vi "configuration UI.vi"() -> ()   [LabVIEW 2013, in "Profibus Module editor node.lvclass"]
uses:
  Profibus Module editor node.lvclass
  <vilib>/NI/Configuration Framework/Node/NodeRef.ctl
  <vilib>/NI/Configuration Framework/Node/NISE_CEF_Node.lvclass
  <vilib>/NI/AMC/Message Queue.ctl
  <vilib>/NI/AMC/Message.ctl
  <vilib>/NI/Tools/Keyed Array/KeyedArray.ctl
  <vilib>/NI/Configuration Framework/Node/UserEventRef.ctl
  <vilib>/NI/Configuration Framework/Controls/EventCluster.ctl
  configuration/endianness setting.ctl
  configuration/error throw specification.ctl
  <vilib>/NI/Tag Bus Data Framework/Configuration Editor/Classes/Engine Parent/Engine Parent Editor Node.lvclass
  <vilib>/NI/Tag Bus/tag/tag descriptor.lvclass
  <vilib>/NI/Tag Bus/tag/Data Type.ctl
  <vilib>/NI/Module Execution Interface/Engine Configuration/engine configuration.lvclass
  <vilib>/NI/Tag Bus/tag/tag descriptor.lvclass/tag descriptor.ctl
  Profibus Module editor node.lvclass/Profibus Module editor node.ctl
  configuration/Profibus Module configuration.lvclass/Profibus Module configuration.ctl
  <vilib>/NI/Configuration Framework/serializable configuration/NISE_CEF_serializable configuration.lvclass/NISE_CEF_serializable configuration.ctl
  configuration/slave diagnostic configuration.ctl
  <vilib>/NI/Tag Bus Module Framework/channel/TBM channel.lvclass
  <vilib>/NI/Tag Bus/tag/write tag name.vi
  <vilib>/NI/Tag Bus/tag/write data type.vi
  configuration/Write RIO interface.vi
  <vilib>/Utility/LVClass/Get LV Class Name.vi
  <vilib>/NI/Configuration Framework/error generator/NISE_error generator.vi
  <vilib>/NI/Configuration Framework/NISE_CEF_TreeControl.lvlib
  configuration/Profibus Module configuration.lvclass
  <vilib>/NI/Tag Bus Data Framework/Configuration Editor/Classes/Module editor node/module editor node.lvclass
  channel/Profibus channel.lvclass
  <vilib>/NI/Configuration Framework/serializable configuration/NISE_CEF_serializable configuration.lvclass
  <vilib>/NI/Tools/Keyed Array/Tools_KeyedArray.lvlib
  <vilib>/NI/AMC/AMC.lvlib
panel:
  in  "Tab Control":T1(tab)
  in  "Remove Button":bool
  in  "Add Button":bool
  in  "channel":i32(listbox)
  in  "settings":bool
  in  "slave":i8
  in  "remove slave":bool
  in  "add slave":bool
  in  "byte order":T2
  out "Configured Order":T2[](array[typedef])
  in  "RIO Interface":string="RIO0"
  in  "Channel Name?":string
  in  "error specs":T3[](array[typedef])
  in  "report?":bool
  out "Selected Slave":i8
  in  "disablediag":bool
  in  "enablediag":bool
  in  "Slaves to Enable Diagnostics":i32(listbox)
  in  "Available Slaves":i32(listbox)
  in  "user event":T4
  in  "main queue":T5
  in  "node ref":T6
  # "Default configuration is little endian"
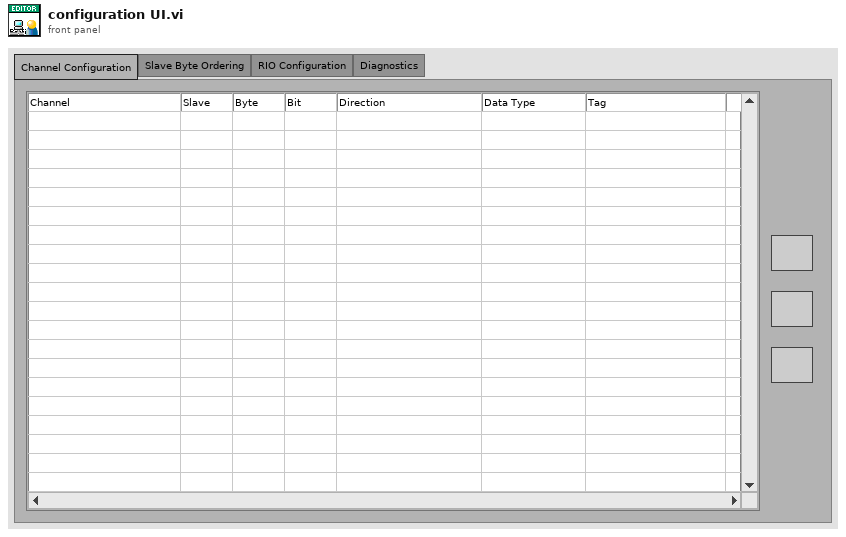
[diagram p1: front panel]
types:
  T1 = enum32{"Channel Configuration", "Slave Byte Ordering", "RIO Configuration", "Diagnostics"}
  T2 = typedef "Profibus Module configuration.lvclass/endianness setting.ctl" = cluster{"slave":i8, "big endian":bool}
  T3 = typedef "Profibus Module configuration.lvclass/error throw specification.ctl" = cluster{"byte":i32, "bit":i32, "inverted?":bool, "error":i32}
  T4 = typedef "NISE_CEF_Node.lvclass/UserEventRef.ctl" = refnum<user-event>
  T5 = typedef "AMC.lvlib/Message Queue.ctl" = refnum<queue>
  T6 = typedef "NISE_CEF_Node.lvclass/NodeRef.ctl" = refnum<data-value>
  T7 = typedef "NISE_CEF_TreeControl.lvlib/EventCluster.ctl" = cluster{"command":string, "data":string}
  T8 = typedef "tag bus.lvlib/tag descriptor.lvclass/Data Type.ctl" = enum16{"Double", "Single", "I64", "I32", "I16", "I8", "U64", "U32", "U16", "U8", "Boolean", "String", "Array of Double", "Array of Single", "Array of I64", "Array of I32", "Array of I16", "Array of I8", "Array of U64", "Array of U32", "Array of U16", "Array of U8", "Array of Boolean", "Array of String"}
  T9 = typedef "Profibus Module configuration.lvclass/slave diagnostic configuration.ctl" = cluster{"slave":i8, "report":bool, "channel":refnum<class "TBM channel.lvclass">, "error specs":T3[]}
  T10 = typedef "Profibus Module editor node.lvclass/table line.ctl" = cluster{"profchan":refnum<class "Profibus channel.lvclass">, "tag name":string}
  T11 = typedef "LVPoint32TypeDef.ctl" = cluster{"Horizontal":i32, "Vertical":i32}
  T12 = typedef "LVRowAndColumnTypeDef.ctl" = cluster{"Row":i32, "Column":i32}
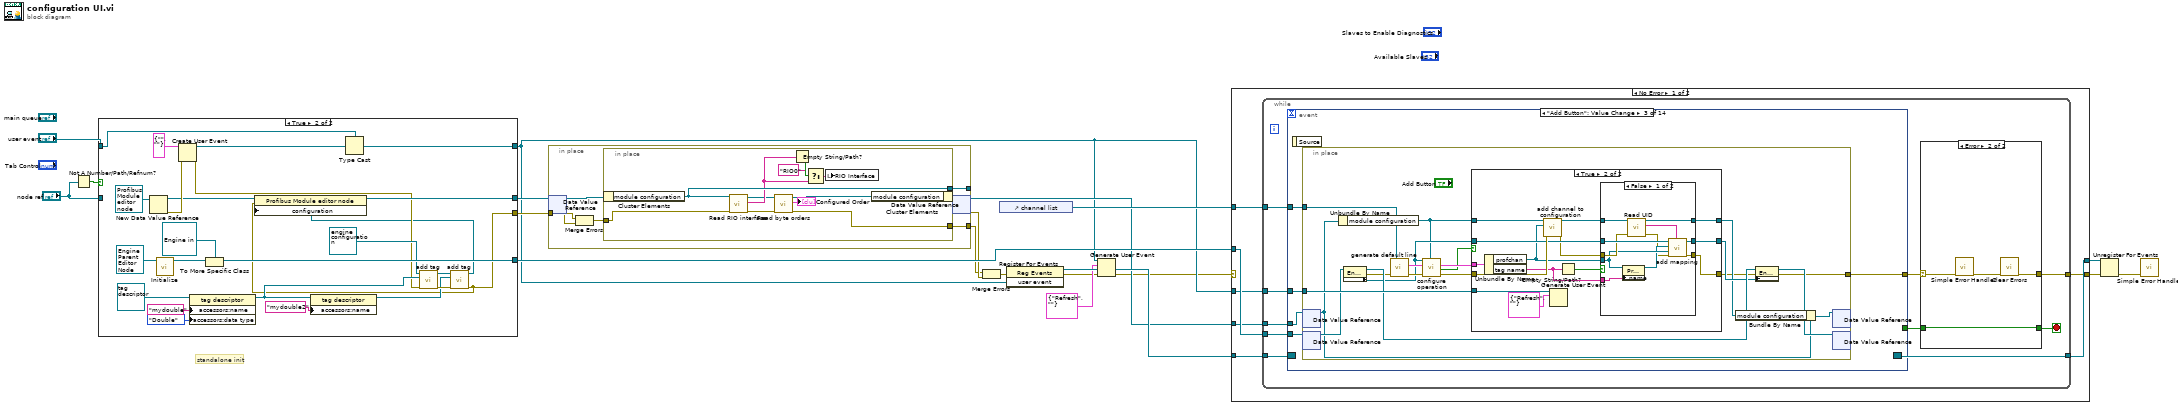
[diagram p0: block diagram]
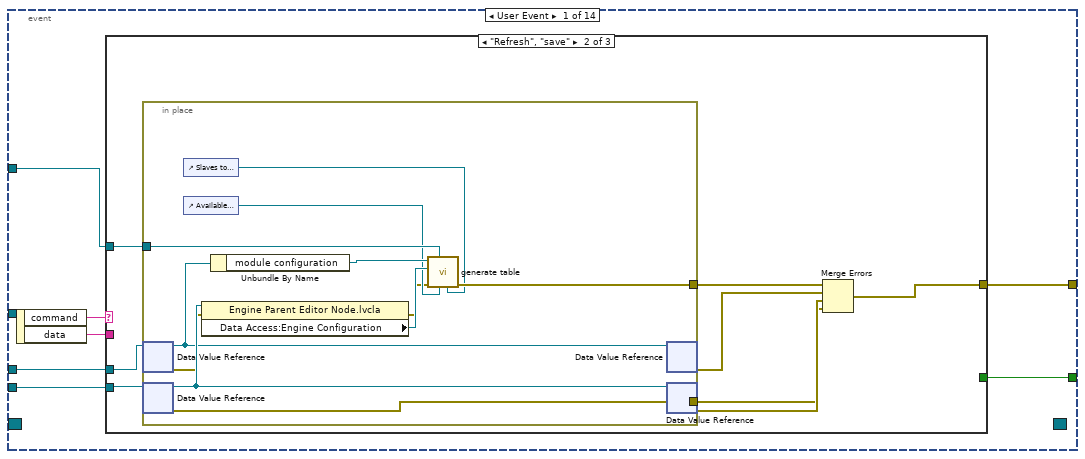
[diagram p3: hidden frame]
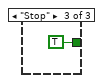
[diagram p5: hidden frame]
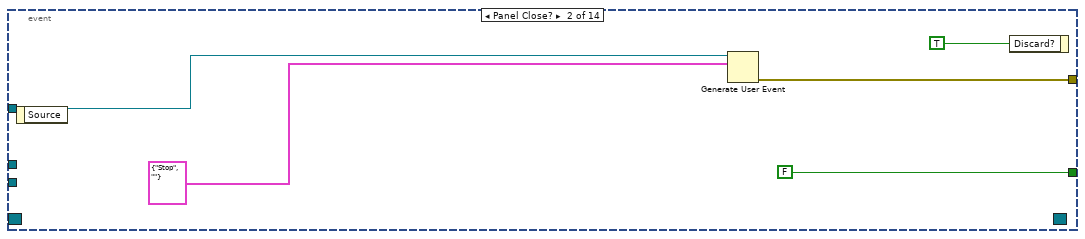
[diagram p6: hidden frame]
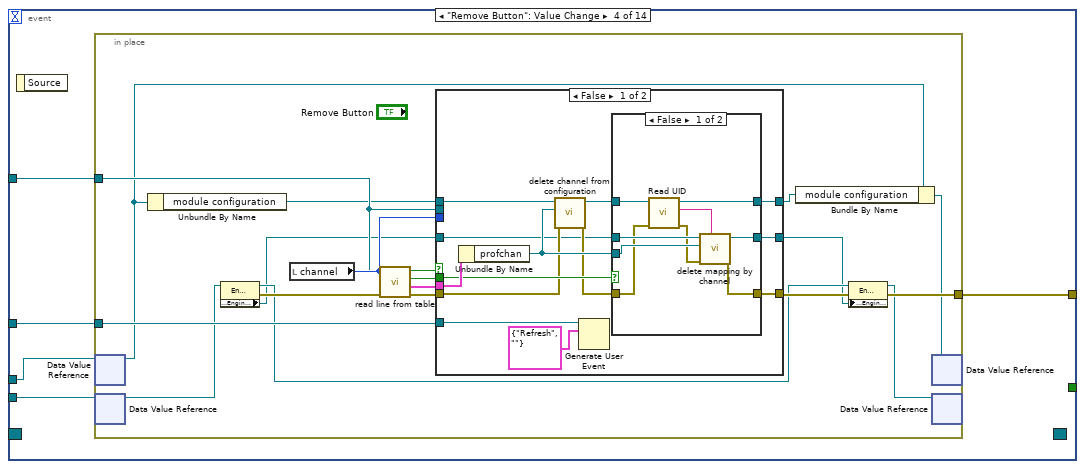
[diagram p9: hidden frame]
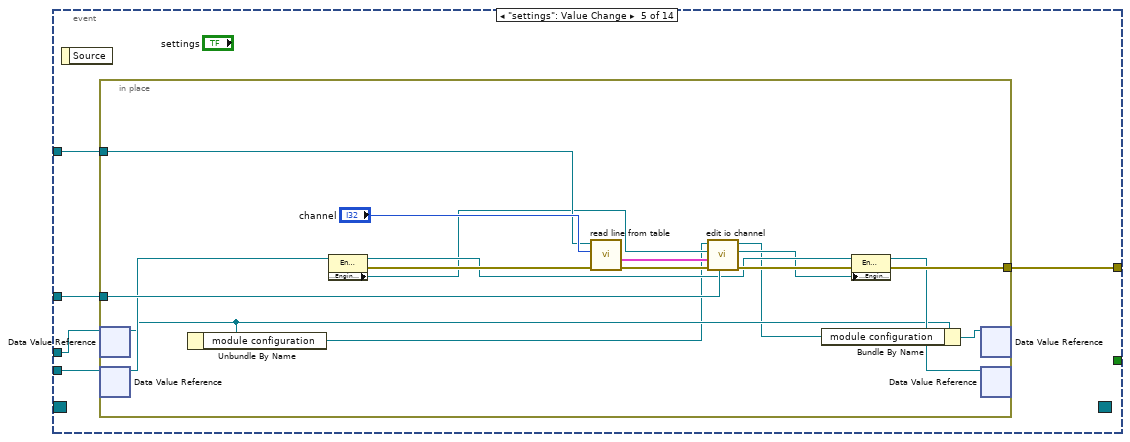
[diagram p12: hidden frame]
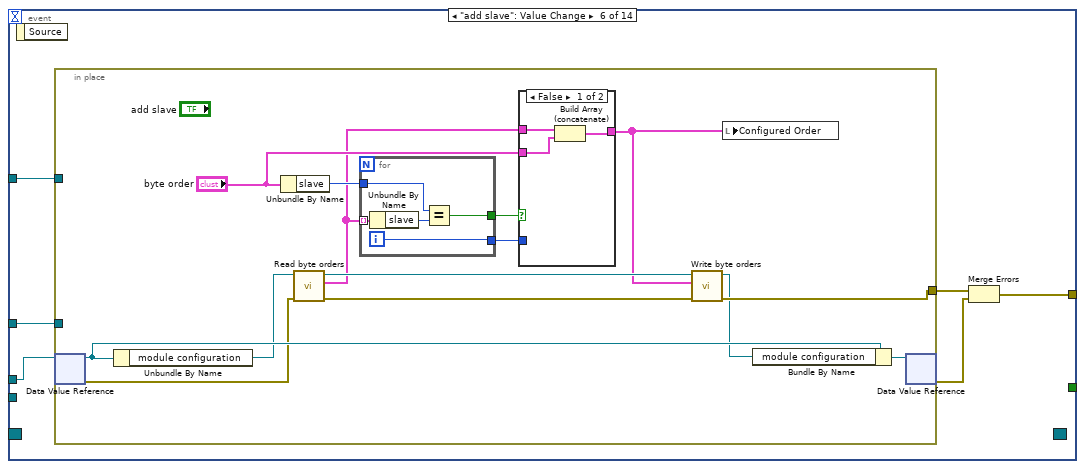
[diagram p13: hidden frame]
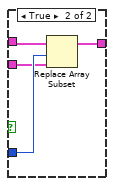
[diagram p14: hidden frame]
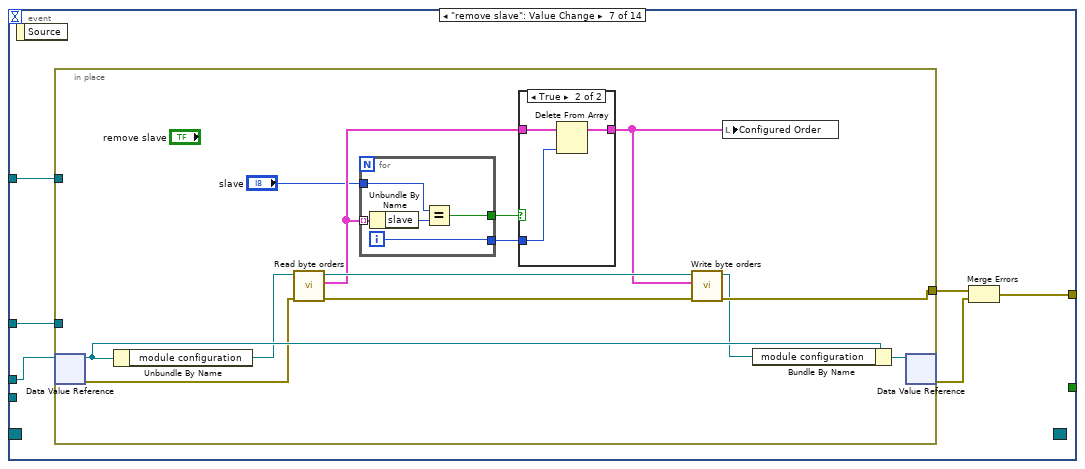
[diagram p15: hidden frame]
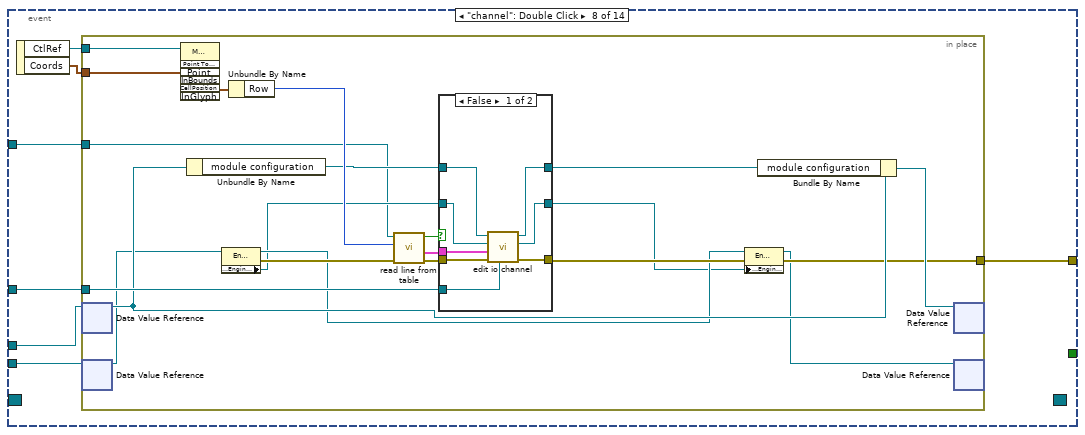
[diagram p17: hidden frame]
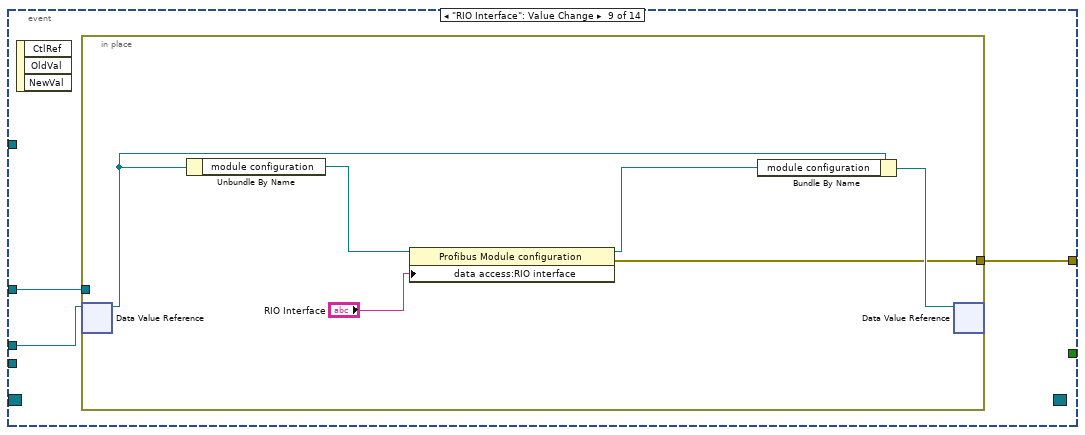
[diagram p19: hidden frame]
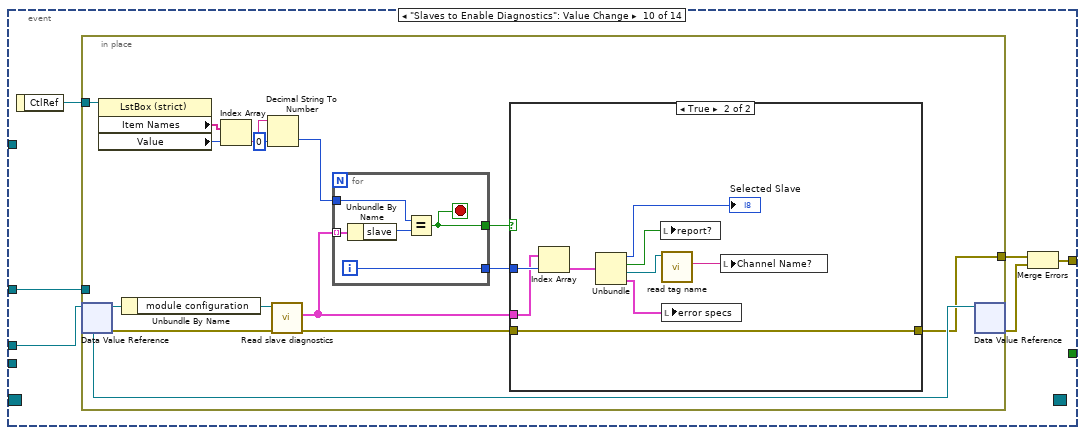
[diagram p20: hidden frame]
diagram:
  # "standalone init"
  n1 = Not A Number/Path/Refnum?(number/path/refnum="node ref") -> (NaN/Path/Refnum?=w16:bool)
  n2 = case shown="True" w16 {
    tunnel: "user event" -> [w26 w31]
    tunnel: [w26 w32] -> w3
    tunnel: "node ref" -> [w24 _]
    tunnel: [w23 w46] -> w10
    tunnel: [w22 w28] -> w9
    tunnel: [w21 w43] -> w14
    frame False {
      n3 = call <vilib>:"locate engine.vi"("component"=w24) -> ("error out"=w20:errorcluster, "engine"=w21:refnum<data-value>)  [unwired: 9 in]
      n4 = To More Specific Class(target class=refnum<data-value> refnum ("data value reference"), reference=w24, error in=w20) -> (specific class reference=w23:refnum<data-value>, error out=w22:errorcluster)
    }
    frame True {
      n5 = New Data Value Reference(data value=refnum<class "Profibus Module editor node.lvclass"> refnum ("tag bus configurable plugin editor node")) -> (data value reference=w45:refnum<data-value>, error out=w47:errorcluster)  [unwired: 1 in]
      n6 = call-dynamic "Initialize.vi"("Engine in"=refnum<class "Engine Parent Editor Node.lvclass"> refnum) -> ("data value reference"=w44:T6)  [unwired: 8 in, 2 out]
      n7 = Create User Event(user event datatype=T7 {"command"="", "data"=""} ("event data"), error in=w47) -> (user event=w49:refnum<user-event>, error out=w29:errorcluster)
      n8 = property class="tag descriptor"(reference=refnum<class "tag descriptor.lvclass"> refnum ("tag descriptor"), "accessors:name"="mydouble" ("name"), "accessors:data type"=Data_Type."Double" ("data type")) -> (reference out=w33:refnum<class "tag descriptor.lvclass">)  [unwired: 1 in, 1 out]
      n9 = To More Specific Class(target class=refnum<data-value> refnum ("data value reference"), reference=w44) -> (specific class reference=w43:refnum<data-value>)  [unwired: 1 in, 1 out]
      n10 = property class="tag descriptor"(reference=w33, "accessors:name"="mydouble2" ("name")) -> (reference out=w34:refnum<class "tag descriptor.lvclass">)  [unwired: 1 in, 1 out]
      n11 = Type Cast(type=w31, x=w49) -> (*(type *) &x=w32:T4)
      n12 = call <vilib>:"add tag.vi"("error in"=w29, "tag descriptor"=w33, "engine configuration in"=refnum<class "engine configuration.lvclass"> refnum ("Engine Configuration")) -> ("error out"=w36:errorcluster, "engine configuration out"=w35:refnum<class "engine configuration.lvclass">)  [unwired: 7 in]
      n13 = call <vilib>:"add tag.vi"("error in"=w36, "tag descriptor"=w34, "engine configuration in"=w35) -> ("error out"=w28:errorcluster, "engine configuration out"=w27:refnum<class "engine configuration.lvclass">)  [unwired: 7 in]
      n14 = property class="Profibus Module editor node"(reference=w45, error in=w28, "configuration"=w27) -> (reference out=w46:refnum<data-value>)  [unwired: 1 out]
    }
  }
  n15 = in-place {
    in-place-border: w9 -> [w57]
    in-place-border: [w52] -> w7
    in-place-border: [w51] -> _
    n16 = in-place-dvr #1(w10) -> (w55:refnum<class "Profibus Module editor node.lvclass">, w56:errorcluster)
    n17 = Merge Errors(w57, w56) -> (w53:errorcluster)
    n18 = in-place {
      in-place-border: w53 -> [w67]
      in-place-border: [w60] -> w52
      in-place-border: [w68] -> w51
      n19 = in-place-cluster #2(w55) -> ("module configuration"=w68:refnum<class "Profibus Module configuration.lvclass">)
      n20 = call "Read RIO interface.vi"("error in"=w67, "Profibus Module configuration in"=w68) -> ("error out"=w59:errorcluster, "RIO interface"=w63:string, "Profibus Module configuration out"=w62:refnum<class "Profibus Module configuration.lvclass">)  [unwired: 7 in]
      n21 = call "Read byte orders.vi"("error in"=w59, "Profibus Module configuration in"=w62) -> ("error out"=w60:errorcluster, "byte orders"=→"Configured Order":T2[], "Profibus Module configuration out"=w61:refnum<class "Profibus Module configuration.lvclass">)  [unwired: 7 in]
      n22 = Empty String/Path?(string/path=w63) -> (empty?=w66:bool)
      n23 = Select(t="RIO0", s=w66, f=w63) -> (s? t:f=w64:string)
      n24 = local write "RIO Interface"(w64) -> ()
      n25 = in-place-cluster #2("module configuration"=w61) -> (w54:refnum<class "Profibus Module editor node.lvclass">)
    }
    n26 = in-place-dvr #1(w54) -> (w6:refnum<data-value>, w8:errorcluster)
  }
  n27 = Merge Errors(w7, w8) -> (w5:errorcluster)
  n28 = control-ref of="channel list"() -> (w12:refnum<vi>)
  n29 = register-events(error in=w5, w3) -> (reference out=w19:refnum<event-registration>, error out=w2:errorcluster)  [unwired: 1 in]
  n30 = Generate User Event(user event=w3, event data cluster=T7 {"command"="Refresh", "data"=""} ("event data"), error in=w2) -> (error out=w1:errorcluster)  [unwired: 1 in, 1 out]
  n31 = case shown="No Error" w1 {
    selector: w1 -> [_ w546]
    tunnel: w19 -> [w75 w545]
    tunnel: [w74 w545] -> w18
    tunnel: [w73 w546] -> w17
    tunnel: w14 -> [w72 _]
    tunnel: w12 -> [w71 _]
    tunnel: w6 -> [w70 _]
    tunnel: w3 -> [w69 _]
    frame No Error {
      n32 = while {
        tunnel: w75 -> [w85]
        tunnel: [w84] -> w74
        tunnel: w70 -> [w81]
        tunnel: w72 -> [w80]
        tunnel: w69 -> [w79]
        tunnel: w71 -> [w77]
        tunnel: [w82] -> w73
        stop <- w83 stop-if-true
        n33 = event shown="[2] \"Add Button\": Value Change" {
          selector: w85 -> [_ _ _ _ _ _ _ _ _ _ _ _ _ _]
          dyn-events: [_ _ _ _ _ _ _ _ _ _ _ _ _ _] -> w84
          timeout: _ -> [_ _ _ _ _ _ _ _ _ _ _ _ _ _]
          tunnel: [w98 FALSE _ _ _ _ _ _ _ _ _ _ _ _] -> w76
          tunnel: [w93 w119 w128 w183 w234 w255 w287 w319 w354 w363 w405 w431 w467 w504] -> w78
          tunnel: w81 -> [w96 _ w124 w179 w231 w256 w288 w314 w352 w365 w406 w432 w470 w507]
          tunnel: w80 -> [w95 _ w125 w180 w232 _ _ w315 _ _ w402 _ _ _]
          tunnel: w79 -> [_ w121 w127 w182 w235 w258 w290 w318 w353 w366 w407 w433 w471 w508]
          tunnel: w77 -> [w92 _ w126 w181 w233 w257 w289 w313 _ _ _ _ _ _]
          event User Event {
            n34 = event-data() -> ("command"=w97:string, "data"=w94:string)  [unwired: 1 in]
            n35 = case shown="\"Refresh\", \"save\"" w97 {
              tunnel: [_ _ TRUE] -> w98
              tunnel: w96 -> [_ w103 _]
              tunnel: w95 -> [_ w104 _]
              tunnel: w94 -> [_ _ _]
              tunnel: [_ w102 _] -> w93
              tunnel: w92 -> [_ w105 _]
              frame Default {
              }
              frame "Refresh", "save" {
                n36 = in-place {
                  in-place-border: [w117] -> w106
                  in-place-border: w105 -> [w116]
                  in-place-border: [w107] -> w99
                  n37 = in-place-dvr #3(w103) -> (w112:refnum<class "Profibus Module editor node.lvclass">, w108:errorcluster)
                  n38 = in-place-dvr #4(w104) -> (w113:refnum<class "Engine Parent Editor Node.lvclass">, w107:errorcluster)
                  n39 = control-ref of="Slaves to Enable Diagnostics"() -> (w111:refnum<vi>)
                  n40 = control-ref of="Available Slaves"() -> (w110:refnum<vi>)
                  n41 = property class="Engine Parent Editor Node.lvcla"(reference=w113, error in=w108) -> (error out=w109:errorcluster, "Data Access:Engine Configuration"=w114:refnum<class "engine configuration.lvclass">)  [unwired: 1 out]
                  n42 = Unbundle By Name(w112) -> ("module configuration"=w115:refnum<class "Profibus Module configuration.lvclass">)
                  n43 = call "generate table.vi"("Slaves to Enable Diagnostics"=w111, "Available Slaves"=w110, "table"=w116, "error in"=w109, "engine configuration in"=w114, "Profibus Module configuration in"=w115) -> ("error out"=w117:errorcluster)  [unwired: 5 in]
                  n44 = in-place-dvr #3(w112) -> (w101:errorcluster)  [unwired: 1 out]
                  n45 = in-place-dvr #4(w113) -> (w100:errorcluster)  [unwired: 1 out]
                }
                n46 = Merge Errors(w106, w101, w100, w99) -> (w102:errorcluster)
              }
              frame "Stop" {
              }
            }
          }
          event Panel Close? {
            n47 = event-data() -> ()  [unwired: 1 in, 1 out]
            n48 = Generate User Event(user event=w121, event data cluster=T7 {"command"="Stop", "data"=""} ("event data")) -> (error out=w119:errorcluster)  [unwired: 2 in, 1 out]
            n49 = event-data("Discard?"=TRUE) -> ()  [unwired: 1 in, 1 out]
          }
          event "Add Button": Value Change {
            n50 = event-data() -> ()  [unwired: 1 in, 1 out]
            n51 = in-place {
              in-place-border: [w129] -> w128
              in-place-border: w127 -> [w142]
              in-place-border: w126 -> [w141]
              n52 = in-place-dvr #5(w124) -> (w135:refnum<class "Profibus Module editor node.lvclass">)  [unwired: 1 out]
              n53 = in-place-dvr #6(w125) -> (w140:refnum<class "Engine Parent Editor Node.lvclass">)  [unwired: 1 out]
              n54 = Unbundle By Name(w135) -> ("module configuration"=w134:refnum<class "Profibus Module configuration.lvclass">)
              n55 = property class="Engine Parent Editor Node.lvcla"(reference=w140) -> (reference out=w138:refnum<class "Engine Parent Editor Node.lvclass">, error out=w131:errorcluster, "Data Access:Engine Configuration"=w136:refnum<class "engine configuration.lvclass">)  [unwired: 1 in]
              n56 = call "generate default line.vi"("error in"=w131, "operations table"=w141) -> ("error out"=w146:errorcluster, "line"=w147:T10)  [unwired: 8 in]
              n57 = call "configure operation.vi"("owner ID"=w134, "error in"=w146, "line item in"=w147, "engine configuration in"=w136) -> ("error out"=w144:errorcluster, "success"=w143:bool, "line item out"=w145:T10)  [unwired: 4 in, 1 out]
              n58 = case shown="True" w143 {
                tunnel: [w150 w153] -> w130
                tunnel: w144 -> [w150 w162]
                tunnel: w136 -> [w149 w160]
                tunnel: w145 -> [_ w163]
                tunnel: w134 -> [w148 w164]
                tunnel: [w149 w159] -> w137
                tunnel: [w148 w154] -> w132
                tunnel: w142 -> [_ w152]
                frame False {
                }
                frame True {
                  n59 = Unbundle By Name(w163) -> ("profchan"=w157:refnum<class "Profibus channel.lvclass">, "tag name"=w156:string)
                  n60 = call "add channel to configuration.vi"("error in"=w162, "TBM channel in"=w157, "Profibus Module configuration in"=w164) -> ("error out"=w158:errorcluster, "Profibus Module configuration out"=w155:refnum<class "Profibus Module configuration.lvclass">)  [unwired: 7 in]
                  n61 = Generate User Event(user event=w152, event data cluster=T7 {"command"="Refresh", "data"=""} ("event data")) -> ()  [unwired: 2 in, 2 out]
                  n62 = Empty String/Path?(string/path=w156) -> (empty?=w161:bool)
                  n63 = case shown="False" w161 {
                    tunnel: w160 -> [w175 w178]
                    tunnel: [w174 w178] -> w159
                    tunnel: w158 -> [w173 w177]
                    tunnel: w157 -> [w172 _]
                    tunnel: w156 -> [w171 _]
                    tunnel: [w169 w177] -> w153
                    tunnel: w155 -> [w167 w176]
                    tunnel: [w166 w176] -> w154
                    frame False {
                      n64 = property class="Profibus channel.lvclass"(reference=w172, "accessors:name"=w171) -> (reference out=w170:refnum<class "Profibus channel.lvclass">)  [unwired: 1 in, 1 out]
                      n65 = call <vilib>:"Read UID.vi"("error in"=w173, "configuration in"=w167) -> ("error out"=w168:errorcluster, "instance id"=w165:string, "configuration out"=w166:refnum<class "Profibus Module configuration.lvclass">)  [unwired: 7 in]
                      n66 = call <vilib>:"add mapping.vi"("owner ID"=w165, "error in"=w168, "channel"=w172, "tag descriptor"=w170, "engine configuration"=w175) -> ("error out"=w169:errorcluster, "engine configuration out"=w174:refnum<class "engine configuration.lvclass">)  [unwired: 5 in]
                    }
                    frame True {
                    }
                  }
                }
              }
              n67 = Bundle By Name(cluster=w135, "module configuration"=w132) -> (w133:refnum<class "Profibus Module editor node.lvclass">)
              n68 = property class="Engine Parent Editor Node.lvcla"(reference=w138, error in=w130, "Data Access:Engine Configuration"=w137) -> (reference out=w139:refnum<class "Engine Parent Editor Node.lvclass">, error out=w129:errorcluster)
              n69 = in-place-dvr #5(w133) -> ()  [unwired: 2 out]
              n70 = in-place-dvr #6(w139) -> ()  [unwired: 2 out]
            }
          }
          event "Remove Button": Value Change {
            n71 = event-data() -> ()  [unwired: 1 in, 1 out]
            n72 = in-place {
              in-place-border: [w193] -> w183
              in-place-border: w182 -> [w196]
              in-place-border: w181 -> [w195]
              n73 = in-place-dvr #7(w179) -> (w186:refnum<class "Profibus Module editor node.lvclass">)  [unwired: 1 out]
              n74 = in-place-dvr #8(w180) -> (w191:refnum<class "Engine Parent Editor Node.lvclass">)  [unwired: 1 out]
              n75 = Unbundle By Name(w186) -> ("module configuration"=w187:refnum<class "Profibus Module configuration.lvclass">)
              n76 = property class="Engine Parent Editor Node.lvcla"(reference=w191) -> (reference out=w192:refnum<class "Engine Parent Editor Node.lvclass">, error out=w194:errorcluster, "Data Access:Engine Configuration"=w189:refnum<class "engine configuration.lvclass">)  [unwired: 1 in]
              n77 = local read "channel"() -> (w201:i32)
              n78 = call "read line from table.vi"("error in"=w194, "line number"=w201, "channels table"=w195) -> ("error out"=w197:errorcluster, "line"=w200:T10, "empty tag?"=w198:bool, "empty channel?"=w199:bool)  [unwired: 5 in]
              n79 = case shown="False" w199 {
                tunnel: [w205 w229] -> w202
                tunnel: w201 -> [_ _]
                tunnel: w195 -> [_ _]
                tunnel: w200 -> [w215 _]
                tunnel: w187 -> [w213 w228]
                tunnel: w189 -> [w208 w230]
                tunnel: w198 -> [w214 _]
                tunnel: w197 -> [w211 w229]
                tunnel: [w207 w230] -> w188
                tunnel: [w206 w228] -> w184
                tunnel: w196 -> [w203 _]
                frame False {
                  n80 = Unbundle By Name(w215) -> ("profchan"=w212:refnum<class "Profibus channel.lvclass">)
                  n81 = call "delete channel from configuration.vi"("error in"=w211, "TBM channel in"=w212, "Profibus Module configuration in"=w213) -> ("error out"=w209:errorcluster, "Profibus Module configuration out"=w210:refnum<class "Profibus Module configuration.lvclass">)  [unwired: 7 in]
                  n82 = Generate User Event(user event=w203, event data cluster=T7 {"command"="Refresh", "data"=""} ("event data")) -> ()  [unwired: 2 in, 2 out]
                  n83 = case shown="False" w214 {
                    tunnel: w212 -> [w223 _]
                    tunnel: w210 -> [w218 w225]
                    tunnel: w209 -> [w222 w226]
                    tunnel: w208 -> [w224 w227]
                    tunnel: [w221 w227] -> w207
                    tunnel: [w220 w226] -> w205
                    tunnel: [w217 w225] -> w206
                    frame False {
                      n84 = call <vilib>:"Read UID.vi"("error in"=w222, "configuration in"=w218) -> ("error out"=w219:errorcluster, "instance id"=w216:string, "configuration out"=w217:refnum<class "Profibus Module configuration.lvclass">)  [unwired: 7 in]
                      n85 = call <vilib>:"delete mapping by channel.vi"("owner ID"=w216, "error in"=w219, "channel"=w223, "engine configuration in"=w224) -> ("error out"=w220:errorcluster, "engine configuration out"=w221:refnum<class "engine configuration.lvclass">)  [unwired: 6 in]
                    }
                    frame True {
                    }
                  }
                }
                frame True {
                }
              }
              n86 = Bundle By Name(cluster=w186, "module configuration"=w184) -> (w185:refnum<class "Profibus Module editor node.lvclass">)
              n87 = property class="Engine Parent Editor Node.lvcla"(reference=w192, error in=w202, "Data Access:Engine Configuration"=w188) -> (reference out=w190:refnum<class "Engine Parent Editor Node.lvclass">, error out=w193:errorcluster)
              n88 = in-place-dvr #7(w185) -> ()  [unwired: 2 out]
              n89 = in-place-dvr #8(w190) -> ()  [unwired: 2 out]
            }
          }
          event "settings": Value Change {
            n90 = event-data() -> ()  [unwired: 1 in, 1 out]
            n91 = in-place {
              in-place-border: w235 -> [w250]
              in-place-border: [w245] -> w234
              in-place-border: w233 -> [w247]
              n92 = in-place-dvr #9(w231) -> (w239:refnum<class "Profibus Module editor node.lvclass">)  [unwired: 1 out]
              n93 = in-place-dvr #10(w232) -> (w242:refnum<class "Engine Parent Editor Node.lvclass">)  [unwired: 1 out]
              n94 = Unbundle By Name(w239) -> ("module configuration"=w238:refnum<class "Profibus Module configuration.lvclass">)
              n95 = property class="Engine Parent Editor Node.lvcla"(reference=w242) -> (reference out=w244:refnum<class "Engine Parent Editor Node.lvclass">, error out=w246:errorcluster, "Data Access:Engine Configuration"=w240:refnum<class "engine configuration.lvclass">)  [unwired: 1 in]
              n96 = call "read line from table.vi"("error in"=w246, "line number"="channel", "channels table"=w247) -> ("error out"=w252:errorcluster, "line"=w251:T10)  [unwired: 5 in, 2 out]
              n97 = call "edit io channel.vi"("user event"=w250, "error in"=w252, "line"=w251, "engine configuration in"=w240, "Profibus Module configuration in"=w238) -> ("error out"=w249:errorcluster, "engine configuration out"=w241:refnum<class "engine configuration.lvclass">, "Profibus Module configuration out"=w237:refnum<class "Profibus Module configuration.lvclass">)  [unwired: 4 in]
              n98 = Bundle By Name(cluster=w239, "module configuration"=w237) -> (w236:refnum<class "Profibus Module editor node.lvclass">)
              n99 = property class="Engine Parent Editor Node.lvcla"(reference=w244, error in=w249, "Data Access:Engine Configuration"=w241) -> (reference out=w243:refnum<class "Engine Parent Editor Node.lvclass">, error out=w245:errorcluster)
              n100 = in-place-dvr #9(w236) -> ()  [unwired: 2 out]
              n101 = in-place-dvr #10(w243) -> ()  [unwired: 2 out]
            }
          }
          event "add slave": Value Change {
            n102 = event-data() -> ()  [unwired: 1 in, 1 out]
            n103 = in-place {
              in-place-border: w258 -> [_]
              in-place-border: w257 -> [_]
              in-place-border: [w268] -> w254
              n104 = in-place-dvr #11(w256) -> (w272:refnum<class "Profibus Module editor node.lvclass">, w270:errorcluster)
              n105 = Unbundle By Name(w272) -> ("module configuration"=w265:refnum<class "Profibus Module configuration.lvclass">)
              n106 = Unbundle By Name("byte order") -> ("slave"=w264:i8)
              n107 = call "Read byte orders.vi"("error in"=w270, "Profibus Module configuration in"=w265) -> ("error out"=w269:errorcluster, "byte orders"=w261:T2[], "Profibus Module configuration out"=w266:refnum<class "Profibus Module configuration.lvclass">)  [unwired: 7 in]
              n108 = for {
                tunnel: w261 -> [w284] mode=indexing
                tunnel: w264 -> [w282]
                tunnel: [w281] -> w263
                tunnel: [w280] -> w260
                i -> [w280]
                n109 = Unbundle By Name(w284) -> ("slave"=w283:i8)
                n110 = Equal?(x=w282, y=w283) -> (x = y?=w281:bool)
              }
              n111 = case shown="False" w263 {
                tunnel: "byte order" -> [w273 w277]
                tunnel: w261 -> [w275 w279]
                tunnel: w260 -> [_ w278]
                tunnel: [w274 w276] -> w259
                frame False {
                  n112 = Build Array (concatenate)(w275, w273) -> (w274:T2[])
                }
                frame True {
                  n113 = Replace Array Subset(array=w279, new element=w277, index=w278) -> (w276:T2[])
                }
              }
              n114 = call "Write byte orders.vi"("error in"=w269, "byte orders"=w259, "Profibus Module configuration in"=w266) -> ("error out"=w268:errorcluster, "Profibus Module configuration out"=w267:refnum<class "Profibus Module configuration.lvclass">)  [unwired: 7 in]
              n115 = local write "Configured Order"(w259) -> ()
              n116 = Bundle By Name(cluster=w272, "module configuration"=w267) -> (w271:refnum<class "Profibus Module editor node.lvclass">)
              n117 = in-place-dvr #11(w271) -> (w253:errorcluster)  [unwired: 1 out]
            }
            n118 = Merge Errors(w254, w253) -> (w255:errorcluster)
          }
          event "remove slave": Value Change {
            n119 = event-data() -> ()  [unwired: 1 in, 1 out]
            n120 = in-place {
              in-place-border: w290 -> [_]
              in-place-border: w289 -> [_]
              in-place-border: [w299] -> w286
              n121 = in-place-dvr #12(w288) -> (w303:refnum<class "Profibus Module editor node.lvclass">, w301:errorcluster)
              n122 = Unbundle By Name(w303) -> ("module configuration"=w296:refnum<class "Profibus Module configuration.lvclass">)
              n123 = call "Read byte orders.vi"("error in"=w301, "Profibus Module configuration in"=w296) -> ("error out"=w300:errorcluster, "byte orders"=w294:T2[], "Profibus Module configuration out"=w297:refnum<class "Profibus Module configuration.lvclass">)  [unwired: 7 in]
              n124 = for {
                tunnel: w294 -> [w312] mode=indexing
                tunnel: "slave" -> [w310]
                tunnel: [w309] -> w295
                tunnel: [w308] -> w293
                i -> [w308]
                n125 = Unbundle By Name(w312) -> ("slave"=w311:i8)
                n126 = Equal?(x=w310, y=w311) -> (x = y?=w309:bool)
              }
              n127 = case shown="True" w295 {
                tunnel: w294 -> [w304 w307]
                tunnel: w293 -> [_ w305]
                tunnel: [w304 w306] -> w292
                frame False {
                }
                frame True {
                  n128 = Delete From Array(array=w307, index=w305) -> (array with subset deleted=w306:T2[])  [unwired: 1 in, 1 out]
                }
              }
              n129 = call "Write byte orders.vi"("error in"=w300, "byte orders"=w292, "Profibus Module configuration in"=w297) -> ("error out"=w299:errorcluster, "Profibus Module configuration out"=w298:refnum<class "Profibus Module configuration.lvclass">)  [unwired: 7 in]
              n130 = local write "Configured Order"(w292) -> ()
              n131 = Bundle By Name(cluster=w303, "module configuration"=w298) -> (w302:refnum<class "Profibus Module editor node.lvclass">)
              n132 = in-place-dvr #12(w302) -> (w285:errorcluster)  [unwired: 1 out]
            }
            n133 = Merge Errors(w286, w285) -> (w287:errorcluster)
          }
          event "channel": Double Click {
            n134 = event-data() -> ("CtlRef"=w317:refnum<vi>, "Coords"=w316:T11)  [unwired: 1 in]
            n135 = in-place {
              in-place-border: [w327] -> w319
              in-place-border: w318 -> [w337]
              in-place-border: w317 -> [w336]
              in-place-border: w316 -> [w335]
              in-place-border: w313 -> [w320]
              n136 = in-place-dvr #13(w314) -> (w331:refnum<class "Profibus Module editor node.lvclass">)  [unwired: 1 out]
              n137 = in-place-dvr #14(w315) -> (w325:refnum<class "Engine Parent Editor Node.lvclass">)  [unwired: 1 out]
              n138 = invoke class="MCListbox (strict)" method="Point To Row Column"(reference=w336, "Point"=w335) -> ("CellPosition"=w334:T12)  [unwired: 5 in, 6 out]
              n139 = Unbundle By Name(w331) -> ("module configuration"=w328:refnum<class "Profibus Module configuration.lvclass">)
              n140 = property class="Engine Parent Editor Node.lvcla"(reference=w325) -> (reference out=w324:refnum<class "Engine Parent Editor Node.lvclass">, error out=w326:errorcluster, "Data Access:Engine Configuration"=w323:refnum<class "engine configuration.lvclass">)  [unwired: 1 in]
              n141 = Unbundle By Name(w334) -> ("Row"=w333:i32)
              n142 = call "read line from table.vi"("error in"=w326, "line number"=w333, "channels table"=w320) -> ("error out"=w339:errorcluster, "line"=w338:T10, "empty channel?"=w332:bool)  [unwired: 5 in, 1 out]
              n143 = case shown="False" w332 {
                tunnel: [w348 w349] -> w340
                tunnel: w339 -> [w347 w349]
                tunnel: w338 -> [w346 _]
                tunnel: w323 -> [w345 w350]
                tunnel: w328 -> [w344 w351]
                tunnel: [w343 w351] -> w329
                tunnel: [w342 w350] -> w322
                tunnel: w337 -> [w341 _]
                frame False {
                  n144 = call "edit io channel.vi"("user event"=w341, "error in"=w347, "line"=w346, "engine configuration in"=w345, "Profibus Module configuration in"=w344) -> ("error out"=w348:errorcluster, "engine configuration out"=w342:refnum<class "engine configuration.lvclass">, "Profibus Module configuration out"=w343:refnum<class "Profibus Module configuration.lvclass">)  [unwired: 4 in]
                }
                frame True {
                }
              }
              n145 = property class="Engine Parent Editor Node.lvcla"(reference=w324, error in=w340, "Data Access:Engine Configuration"=w322) -> (reference out=w321:refnum<class "Engine Parent Editor Node.lvclass">, error out=w327:errorcluster)
              n146 = Bundle By Name(cluster=w331, "module configuration"=w329) -> (w330:refnum<class "Profibus Module editor node.lvclass">)
              n147 = in-place-dvr #13(w330) -> ()  [unwired: 2 out]
              n148 = in-place-dvr #14(w321) -> ()  [unwired: 2 out]
            }
          }
          event "RIO Interface": Value Change {
            n149 = event-data() -> ()  [unwired: 1 in, 3 out]
            n150 = in-place {
              in-place-border: [w359] -> w354
              in-place-border: w353 -> [_]
              n151 = in-place-dvr #15(w352) -> (w356:refnum<class "Profibus Module editor node.lvclass">)  [unwired: 1 out]
              n152 = Unbundle By Name(w356) -> ("module configuration"=w358:refnum<class "Profibus Module configuration.lvclass">)
              n153 = property class="Profibus Module configuration"(reference=w358, "data access:RIO interface"="RIO Interface") -> (reference out=w357:refnum<class "Profibus Module configuration.lvclass">, error out=w359:errorcluster)  [unwired: 1 in]
              n154 = Bundle By Name(cluster=w356, "module configuration"=w357) -> (w360:refnum<class "Profibus Module editor node.lvclass">)
              n155 = in-place-dvr #15(w360) -> ()  [unwired: 2 out]
            }
          }
          event "Slaves to Enable Diagnostics": Value Change {
            n156 = event-data() -> ("CtlRef"=w364:refnum<vi>)  [unwired: 1 in]
            n157 = in-place {
              in-place-border: w366 -> [_]
              in-place-border: w364 -> [w377]
              in-place-border: [w368] -> w362
              n158 = in-place-dvr #16(w365) -> (w380:refnum<class "Profibus Module editor node.lvclass">, w378:errorcluster)
              n159 = property class="LstBox (strict)"(reference=w377) -> ("Item Names"=w376:string[], "Value"=w375:i32)  [unwired: 1 in, 2 out]
              n160 = Unbundle By Name(w380) -> ("module configuration"=w379:refnum<class "Profibus Module configuration.lvclass">)
              n161 = Index Array(array=w376, index=w375) -> (element=w374:string)
              n162 = Decimal String To Number(string=w374, default (0L)=i8 0 ("default (0 I32)")) -> (number=w372:i8)  [unwired: 1 in, 1 out]
              n163 = call "Read slave diagnostics.vi"("error in"=w378, "Profibus Module configuration in"=w379) -> ("error out"=w371:errorcluster, "slave diagnostics"=w367:T9[])  [unwired: 7 in, 1 out]
              n164 = for {
                tunnel: w367 -> [w399] mode=indexing
                tunnel: w372 -> [w397]
                tunnel: [w396] -> w370
                tunnel: [w395] -> w369
                i -> [w395]
                stop <- w396 stop-if-true
                n165 = Unbundle By Name(w399) -> ("slave"=w398:i8)
                n166 = Equal?(x=w397, y=w398) -> (x = y?=w396:bool)
              }
              n167 = case shown="True" w370 {
                tunnel: w371 -> [w385 w394]
                tunnel: w369 -> [_ w393]
                tunnel: [w385 w394] -> w368
                tunnel: w367 -> [_ w392]
                frame False {
                  # "not found"
                  n168 = local write "Channel Name?"("" ("Channel Name?")) -> ()
                  n169 = local write "error specs"(T3[] [] ("error specs")) -> ()
                  n170 = local write "report?"(FALSE ("report?")) -> ()
                  n171 = local write "Selected Slave"(i8 0 ("Selected Slave")) -> ()
                }
                frame True {
                  n172 = Index Array(array=w392, index=w393) -> (element=w391:T9)
                  n173 = Unbundle(w391) -> ("slave"=→"Selected Slave":i8, "report"=w390:bool, "channel"=w389:refnum<class "TBM channel.lvclass">, "error specs"=w387:T3[])
                  n174 = local write "report?"(w390) -> ()
                  n175 = call <vilib>:"read tag name.vi"("system tag in"=w389) -> ("name"=w388:string)  [unwired: 8 in, 2 out]
                  n176 = local write "error specs"(w387) -> ()
                  n177 = local write "Channel Name?"(w388) -> ()
                }
              }
              n178 = in-place-dvr #16(w380) -> (w361:errorcluster)  [unwired: 1 out]
            }
            n179 = Merge Errors(w362, w361) -> (w363:errorcluster)
          }
          event "report?", "Channel Name?": Value Change {
            n180 = event-data() -> ()  [unwired: 1 in, 1 out]
            n181 = in-place {
              in-place-border: w407 -> [_]
              in-place-border: [w427] -> w404
              in-place-border: [w420] -> w400
              n182 = in-place-dvr #17(w402) -> (w423:refnum<class "Engine Parent Editor Node.lvclass">, w422:errorcluster)
              n183 = in-place-dvr #18(w406) -> (w426:refnum<class "Profibus Module editor node.lvclass">, w428:errorcluster)
              n184 = call <vilib>:"read engine configuration.vi"("error in"=w422, "Engine Parent Editor Node in"=w423) -> ("error out"=w419:errorcluster, "engine configuration"=w417:refnum<class "engine configuration.lvclass">, "Engine Parent Editor Node out"=w418:refnum<class "Engine Parent Editor Node.lvclass">)  [unwired: 7 in]
              n185 = Merge Errors(w419, w428) -> (w424:errorcluster)
              n186 = property on="Slaves to Enable Diagnostics" class="LstBox (strict)"() -> ("Item Names"=w412:string[], "Value"=w411:i32)  [unwired: 2 in, 2 out]
              n187 = Index Array(array=w412, index=w411) -> (element=w410:string)
              n188 = Decimal String To Number(string=w410, default (0L)=-1 ("default (0 I32)")) -> (number=w408:i32)  [unwired: 1 in, 1 out]
              n189 = call "update diagnostic channel.vi"("report?"="report?", "Channel Name?"="Channel Name?", "error in"=w424, "Selected Slave"=w408, "engine configuration in"=w417, "Profibus Module editor node in"=w426) -> ("error out"=w427:errorcluster, "new chan name"=w413:string, "engine configuration out"=w416:refnum<class "engine configuration.lvclass">, "Profibus Module editor node out"=w425:refnum<class "Profibus Module editor node.lvclass">)  [unwired: 2 in]
              n190 = local write "Channel Name?"(w413) -> ()
              n191 = call <vilib>:"write engine configuration.vi"("error in"=w419, "engine configuration"=w416, "Engine Parent Editor Node in"=w418) -> ("error out"=w420:errorcluster, "Engine Parent Editor Node out"=w421:refnum<class "Engine Parent Editor Node.lvclass">)  [unwired: 7 in]
              n192 = in-place-dvr #17(w421) -> (w401:errorcluster)  [unwired: 1 out]
              n193 = in-place-dvr #18(w425) -> (w403:errorcluster)  [unwired: 1 out]
            }
            n194 = Merge Errors(w401, w400, w404, w403) -> (w405:errorcluster)
          }
          event "error specs": Value Change {
            n195 = event-data() -> ()  [unwired: 1 in, 1 out]
            n196 = in-place {
              in-place-border: w433 -> [_]
              in-place-border: [w443] -> w430
              n197 = in-place-dvr #19(w432) -> (w451:refnum<class "Profibus Module editor node.lvclass">, w449:errorcluster)
              n198 = property on="Slaves to Enable Diagnostics" class="LstBox (strict)"() -> ("Item Names"=w438:string[], "Value"=w437:i32)  [unwired: 2 in, 2 out]
              n199 = Unbundle By Name(w451) -> ("module configuration"=w450:refnum<class "Profibus Module configuration.lvclass">)
              n200 = Index Array(array=w438, index=w437) -> (element=w436:string)
              n201 = Decimal String To Number(string=w436, default (0L)=-1 ("default (0 I32)")) -> (number=w434:i32)  [unwired: 1 in, 1 out]
              n202 = call "Read slave diagnostics.vi"("error in"=w449, "Profibus Module configuration in"=w450) -> ("error out"=w448:errorcluster, "slave diagnostics"=w445:T9[], "Profibus Module configuration out"=w439:refnum<class "Profibus Module configuration.lvclass">)  [unwired: 7 in]
              n203 = for {
                tunnel: w445 -> [w466] mode=indexing
                tunnel: w434 -> [w464]
                tunnel: [w463] -> w447
                tunnel: [w462] -> w446
                i -> [w462]
                stop <- w463 stop-if-true
                n204 = Unbundle By Name(w466) -> ("slave"=w465:i8)
                n205 = Equal?(x=w464, y=w465) -> (x = y?=w463:bool)
              }
              n206 = case shown="False" w447 {
                tunnel: w448 -> [w454 w458]
                tunnel: w446 -> [_ w457]
                tunnel: [w454 w458] -> w441
                tunnel: w445 -> [w453 w456]
                tunnel: [w453 w455] -> w440
                frame False {
                  # "not found"
                  n207 = One Button Dialog(message="Please select a slave") -> ()  [unwired: 1 in, 1 out]
                }
                frame True {
                  n208 = in-place {
                    n209 = in-place-array #20(w456, w457) -> (w461:T9)
                    n210 = Bundle By Name(cluster=w461, "error specs"="error specs") -> (w459:T9)
                    n211 = in-place-array #20(w459) -> (w455:T9[])  [unwired: 1 out]
                  }
                }
              }
              n212 = call "Write slave diagnostics.vi"("error in"=w441, "slave diagnostics"=w440, "Profibus Module configuration in"=w439) -> ("error out"=w443:errorcluster, "Profibus Module configuration out"=w442:refnum<class "Profibus Module configuration.lvclass">)  [unwired: 7 in]
              n213 = Bundle(cluster=w451, w442) -> (w444:refnum<class "Profibus Module editor node.lvclass">)
              n214 = in-place-dvr #19(w444) -> (w429:errorcluster)  [unwired: 1 out]
            }
            n215 = Merge Errors(w430, w429) -> (w431:errorcluster)
          }
          event "enablediag": Value Change {
            n216 = event-data() -> ()  [unwired: 1 in, 1 out]
            n217 = in-place {
              in-place-border: w471 -> [_]
              in-place-border: [w472] -> w468
              n218 = in-place-dvr #21(w470) -> (w482:refnum<class "Profibus Module editor node.lvclass">, w479:errorcluster)
              n219 = Unbundle By Name(w482) -> ("module configuration"=w481:refnum<class "Profibus Module configuration.lvclass">)
              n220 = property on="Available Slaves" class="LstBox (strict)"(error in=w479) -> (error out=w476:errorcluster, "Item Names"=w478:string[], "Value"=w477:i32)  [unwired: 1 in, 1 out]
              n221 = Delete From Array(array=w478, index=w477) -> (deleted portion=w473:string, array with subset deleted=w475:string[])  [unwired: 1 in]
              n222 = property on="Available Slaves" class="LstBox (strict)"(error in=w476, "Item Names"=w475) -> (error out=w474:errorcluster)  [unwired: 1 in, 1 out]
              n223 = case shown="Default" w473 {
                selector: w473 -> [_ w486]
                tunnel: w481 -> [w485 w503]
                tunnel: [w485 w501] -> w480
                tunnel: w474 -> [w484 w499]
                tunnel: [w484 w491] -> w472
                frame "" {
                }
                frame Default {
                  n224 = Decimal String To Number(string=w486) -> (number=w494:i32)  [unwired: 2 in, 1 out]
                  n225 = call "Read slave diagnostics.vi"("error in"=w499, "Profibus Module configuration in"=w503) -> ("error out"=w502:errorcluster, "slave diagnostics"=w497:T9[], "Profibus Module configuration out"=w500:refnum<class "Profibus Module configuration.lvclass">)  [unwired: 7 in]
                  n226 = Bundle By Name(cluster=T9 {"slave"=0, "report"=FALSE, "channel"=refnum, "error specs"=[]} ("diagnostics settings"), "slave"=w494) -> (w495:T9)
                  n227 = Build Array (concatenate)(w497, w495) -> (w496:T9[])
                  n228 = control-ref of="Slaves to Enable Diagnostics"() -> (w492:refnum<vi>)
                  n229 = call "Write slave diagnostics.vi"("error in"=w502, "slave diagnostics"=w496, "Profibus Module configuration in"=w500) -> ("error out"=w493:errorcluster, "Profibus Module configuration out"=w501:refnum<class "Profibus Module configuration.lvclass">)  [unwired: 7 in]
                  n230 = property on="Property Node" class="LstBox (strict)"(reference=w492, error in=w493) -> (reference out=w489:refnum<vi>, error out=w490:errorcluster, "Item Names"=w488:string[])
                  n231 = Build Array (concatenate)(w488, w486) -> (w487:string[])
                  n232 = property on="Property Node" class="LstBox (strict)"(reference=w489, error in=w490, "Item Names"=w487) -> (error out=w491:errorcluster)  [unwired: 1 out]
                }
              }
              n233 = Bundle By Name(cluster=w482, "module configuration"=w480) -> (w483:refnum<class "Profibus Module editor node.lvclass">)
              n234 = in-place-dvr #21(w483) -> (w469:errorcluster)  [unwired: 1 out]
            }
            n235 = Merge Errors(w469, w468) -> (w467:errorcluster)
          }
          event "disablediag": Value Change {
            n236 = event-data() -> ()  [unwired: 1 in, 1 out]
            n237 = in-place {
              in-place-border: w508 -> [_]
              in-place-border: [w511] -> w505
              n238 = in-place-dvr #22(w507) -> (w521:refnum<class "Profibus Module editor node.lvclass">, w518:errorcluster)
              n239 = control-ref of="Slaves to Enable Diagnostics"() -> (w509:refnum<vi>)
              n240 = Unbundle By Name(w521) -> ("module configuration"=w520:refnum<class "Profibus Module configuration.lvclass">)
              n241 = property on="Property Node" class="LstBox (strict)"(reference=w509, error in=w518) -> (reference out=w510:refnum<vi>, error out=w515:errorcluster, "Item Names"=w517:string[], "Value"=w516:i32)
              n242 = Delete From Array(array=w517, index=w516) -> (deleted portion=w512:string, array with subset deleted=w514:string[])  [unwired: 1 in]
              n243 = property on="Property Node" class="LstBox (strict)"(reference=w510, error in=w515, "Item Names"=w514) -> (error out=w513:errorcluster)  [unwired: 1 out]
              n244 = case shown="Default" w512 {
                selector: w512 -> [_ w529]
                tunnel: w520 -> [w524 w540]
                tunnel: [w524 w538] -> w519
                tunnel: w513 -> [w523 w536]
                tunnel: [w523 w534] -> w511
                frame "" {
                }
                frame Default {
                  n245 = Decimal String To Number(string=w529) -> (number=w527:i32)  [unwired: 2 in, 1 out]
                  n246 = call "Read slave diagnostics.vi"("error in"=w536, "Profibus Module configuration in"=w540) -> ("error out"=w539:errorcluster, "slave diagnostics"=w526:T9[], "Profibus Module configuration out"=w537:refnum<class "Profibus Module configuration.lvclass">)  [unwired: 7 in]
                  n247 = for {
                    tunnel: w527 -> [w543]
                    tunnel: w526 -> [w542] mode=indexing
                    tunnel: [w542] -> w525 mode=indexing if=w541
                    n248 = Unbundle By Name(w542) -> ("slave"=w544:i8)
                    n249 = Not Equal?(x=w543, y=w544) -> (x != y?=w541:bool)
                  }
                  n250 = call "Write slave diagnostics.vi"("error in"=w539, "slave diagnostics"=w525, "Profibus Module configuration in"=w537) -> ("error out"=w535:errorcluster, "Profibus Module configuration out"=w538:refnum<class "Profibus Module configuration.lvclass">)  [unwired: 7 in]
                  n251 = control-ref of="Available Slaves"() -> (w528:refnum<vi>)
                  n252 = property on="Property Node" class="LstBox (strict)"(reference=w528, error in=w535) -> (reference out=w532:refnum<vi>, error out=w533:errorcluster, "Item Names"=w531:string[])
                  n253 = Build Array (concatenate)(w531, w529) -> (w530:string[])
                  n254 = property on="Property Node" class="LstBox (strict)"(reference=w532, error in=w533, "Item Names"=w530) -> (error out=w534:errorcluster)  [unwired: 1 out]
                }
              }
              n255 = Bundle By Name(cluster=w521, "module configuration"=w519) -> (w522:refnum<class "Profibus Module editor node.lvclass">)
              n256 = in-place-dvr #22(w522) -> (w506:errorcluster)  [unwired: 1 out]
            }
            n257 = Merge Errors(w506, w505) -> (w504:errorcluster)
          }
        }
        n258 = case shown="Error" w78 {
          selector: w78 -> [w86 w90]
          tunnel: [w87 w91] -> w83
          tunnel: w76 -> [w87 w91]
          tunnel: [w86 w88] -> w82
          frame No Error {
          }
          frame Error {
            n259 = call <vilib>:"Simple Error Handler.vi"("error in (no error)"=w90) -> ("error out"=w89:errorcluster)  [unwired: 4 in, 4 out]
            n260 = call <vilib>:"Clear Errors.vi"("error in (no error)"=w89) -> ("error out"=w88:errorcluster)  [unwired: 6 in]
          }
        }
      }
    }
    frame Error {
    }
  }
  n261 = Unregister For Events(event registration refnum=w18, error in=w17) -> (error out=w13:errorcluster)
  n262 = call <vilib>:"Simple Error Handler.vi"("error in (no error)"=w13) -> ()  [unwired: 4 in, 5 out]
